vi "aliveMSG.vi"(1 "input":string, 2 "UDN":string, 3 "type of announce":u16(ring) items=["isRootDevice", "device", "service"]) -> (0 "aliveMSG":string)   [LabVIEW 2010]
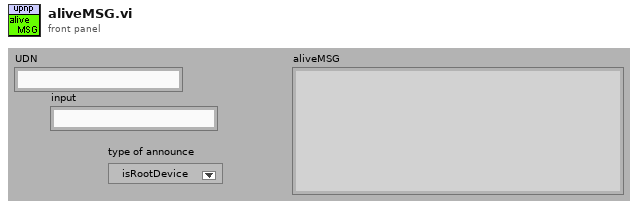
[diagram p1: front panel]
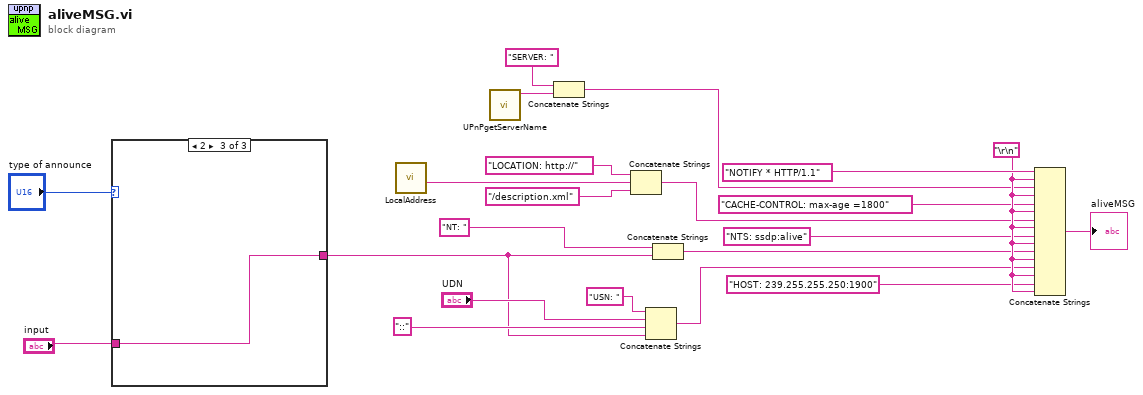
[diagram p0: block diagram]
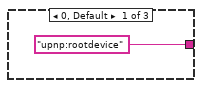
[diagram p2: hidden frame]
diagram:
  w21 = "\r\n"
  n1 = case shown="2" "type of announce" {
    tunnel: ["upnp:rootdevice" w24 w25] -> w6
    tunnel: "input" -> [_ w24 w25]
    frame 0, Default {
    }
    frame 1 {
    }
    frame 2 {
    }
  }
  n2 = call "LocalAddress.vi"() -> ("IP Address (xx.xx.xx.xx)"=w3:string)  [unwired: 11 out]
  n3 = call "UPnPgetServerName.vi"() -> ("ServerName"=w15:string)  [unwired: 11 out]
  n4 = Concatenate Strings("SERVER: " ("string"), w15) -> (w14:string)
  n5 = Concatenate Strings("LOCATION: http://" ("string"), w3, "/description.xml" ("string")) -> (w1:string)
  n6 = Concatenate Strings("USN: " ("string"), "UDN", "::", w6) -> (w9:string)
  n7 = Concatenate Strings("NT: " ("string"), w6) -> (w12:string)
  n8 = Concatenate Strings("NOTIFY * HTTP/1.1" ("string"), w21, w14, w21, "CACHE-CONTROL: max-age =1800" ("string"), w21, w1, w21, "NTS: ssdp:alive" ("string"), w21, w12, w21, w9, w21, "HOST: 239.255.255.250:1900" ("string"), w21) -> (→"aliveMSG":string)
